vi "Run VI Tester Tests.vi"() -> ()   [LabVIEW 2014]
doc: "This VI will execute VI Tester tests.\n\nArguments:\nLabVIEW project file path\nJUnit XML output file path"
uses:
  <vilib>/addons/_JKI.lib/_jki_lib_vi_tester_junit_xml_results.llb/TextTestRunner.JUnitXML.lvclass
  <vilib>/addons/_JKI Toolkits/VI Tester/VI Tester API.llb/Run Tests (Path).vi
  <vilib>/Wiresmith Technology/LabVIEW CLI/CLI Class/CLI.lvclass
  <vilib>/addons/_JKI Toolkits/VI Tester/VI Tester API.llb/VI Tester API.lvlib
panel:
  out "test details":string
  out "error out":errorcluster
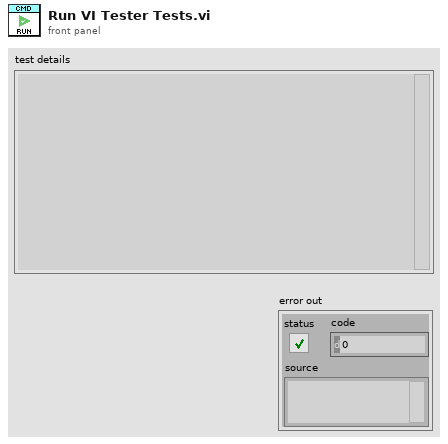
[diagram p1: front panel]
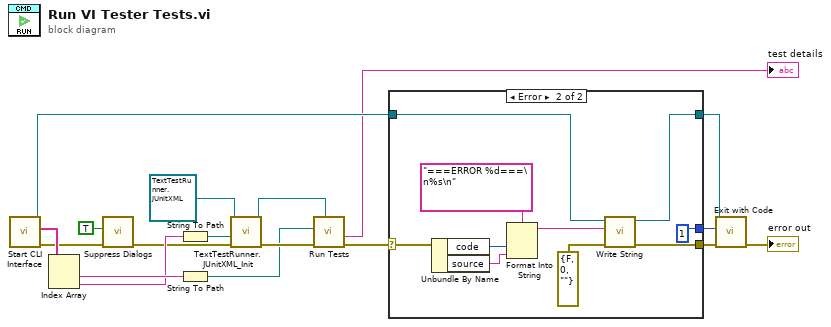
[diagram p0: block diagram]
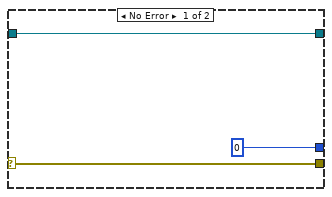
[diagram p2: hidden frame]
diagram:
  n1 = call <vilib>:"Start CLI Interface.vi"() -> ("error out"=w2:errorcluster, "Custom Parameters"=w17:string[], "CLI out"=w14:refnum<class "CLI.lvclass">)  [unwired: 9 in]
  n2 = Index Array(array=w17) -> (element #1=w18:string, element #2=w12:string)  [unwired: 2 in]
  n3 = call "Suppress Dialogs.vi"("error in (no error)"=w2, "Suppress Dialogs? (F)"=TRUE) -> ("error out"=w1:errorcluster)  [unwired: 9 in]
  n4 = String To Path(string=w12) -> (path=w7:path)
  n5 = String To Path(string=w18) -> (path=w6:path)
  n6 = call <vilib>:"TextTestRunner.JUnitXML_Init.vi"("error in (no error)"=w1, "Report Path"=w7, "TextTestRunner in"=refnum<class "TextTestRunner.JUnitXML.lvclass"> refnum ("TextTestRunner.Ant.lvclass")) -> ("error out"=w10:errorcluster, "TextTestRunner out"=w9:refnum<class "TextTestRunner.JUnitXML.lvclass">)  [unwired: 7 in]
  n7 = call-poly <vilib>:"Run Tests.vi"("TextTestRunner in"=w9, "error in (no error)"=w10, "Test Path"=w6) -> ("error out"=w8:errorcluster, "test details"=→"test details":string)  [unwired: 6 in, 1 out]
  n8 = case shown="Error" w8 {
    selector: w8 -> [w21 w28]
    tunnel: w14 -> [w20 w24]
    tunnel: [w21 w27] -> w16
    tunnel: [w20 w26] -> w15
    tunnel: [0 1] -> w13
    frame No Error {
    }
    frame Error {
      n9 = Unbundle By Name(w28) -> ("code"=w29:i32, "source"=w31:string)
      n10 = Format Into String(format string="===ERROR %d===\n%s\n", w29, w31) -> (resulting string=w22:string)  [unwired: 2 in, 1 out]
      n11 = call <vilib>:"Write String.vi"("error in (no error)"=errorcluster {"status"=FALSE, "code"=0, "source"=""} ("error out"), "Text to Write"=w22, "CLI in"=w24) -> ("error out"=w27:errorcluster, "CLI out"=w26:refnum<class "CLI.lvclass">)  [unwired: 7 in]
    }
  }
  n12 = call <vilib>:"Exit with Code.vi"("error in (no error)"=w16, "Exit Code (0)"=w13, "CLI in"=w15) -> ("error out"=→"error out":errorcluster)  [unwired: 8 in]
